vi "ClearReference.vi"(1 "reference in":refnum<class "G#Object.lvclass">) -> (0 "reference out":refnum<class "G#Object.lvclass">)   [LabVIEW 2017, in "G#Object.lvclass"]
doc: "Clears the object reference and makes it invalid.\n\nNotice, this will not delete the object!"
uses:
  G#Object.lvclass
  G#Object.lvclass/G#Object.ctl
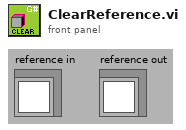
[diagram p1: front panel]
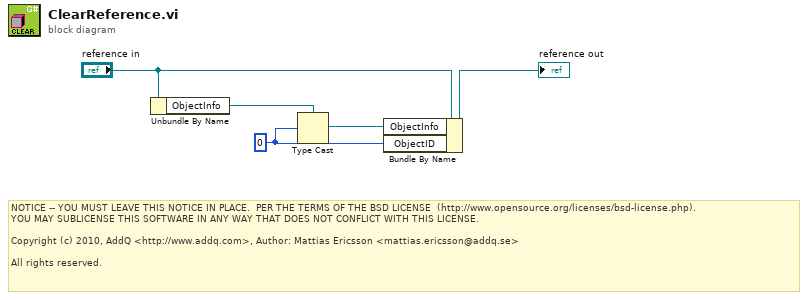
[diagram p0: block diagram]
diagram:
  w1 = u32 0 ("ObjectID")
  # "NOTICE -- YOU MUST LEAVE THIS NOTICE IN PLACE.  PER THE TERMS OF THE BSD LICENSE  (http://www.opensource.org/licenses/bsd-license.php).\nYOU MAY SUBLICENSE THIS SOFTWARE IN ANY WAY THAT DOES NOT CONFLICT WITH THIS LICENSE.\n\nCopyright (c) 2010, AddQ <http://www.addq.com>, Author: Mattias Ericsson <mattias.ericsson@addq.se>\n\nAll rights reserved."
  n1 = Unbundle By Name("reference in") -> ("ObjectInfo"=w5:refnum<queue>)
  n2 = Type Cast(type=w5, x=w1) -> (*(type *) &x=w2:refnum<queue>)
  n3 = Bundle By Name(cluster="reference in", "ObjectInfo"=w2, "ObjectID"=w1) -> (→"reference out":refnum<class "G#Object.lvclass">)
